vi "Drive.vi"() -> ()   [LabVIEW 2012]
uses:
  State_Machine_Enum.ctl
  <vilib>/Rock Robotics/WPI/RobotDrive/WPI_RobotDriveGetSetRefNum.vi
  Robot Global Data.vi
panel:
  out "Loop Difference":u32
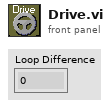
[diagram p1: front panel]
types:
  T1 = typedef "State_Machine_Enum.ctl" = enum16{"Idle", "Start", "Do", "Stop", "Init"}
  T2 = typedef "WPI_RobotDriveDevRef.ctl" = cluster{"DevStatus":errorcluster, "Motors[]":T3[], "Square Inputs":bool, "Max Output":dbl, "Isochronous":bool}
  T3 = typedef "WPI_MotorControlDeviceRef.ctl" = cluster{"DeviceStatus":errorcluster, "Type":enum16{"PWM", "CAN"}, "PWM":cluster{"Digital Module":T4, "PWM Channel":T5, "DeadBand":T6}, "CAN":cluster{"Device Number":u8, "Control Mode":T7, "Semaphore":T8, "Max Vout":dbl}, "Invert":bool, "TransformRef":T9, "InvTransformRef":T9}
  T4 = typedef "FPGA_TypedefDigitalModule.ctl" = enum16{"Digital Module 1", "Digital Module 2"}
  T5 = typedef "FPGA_DIOPWMChannel.ctl" = enum8{"PWM 1", "PWM 2", "PWM 3", "PWM 4", "PWM 5", "PWM 6", "PWM 7", "PWM 8", "PWM 9", "PWM 10", "Invalid"}
  T6 = typedef "WPI_PWMDeadband.ctl" = cluster{"Name":string, "maxPositivePwm":i32, "minPositivePwm":i32, "centerPwm":i32, "maxNegativePwm":i32, "minNegativePwm":i32, "angularRange":u16}
  T7 = typedef "WPI_CANJaguar_ControlMode.ctl" = enum8{"Percent VBus", "Current", "Speed", "Position", "Voltage"}
  T8 = typedef "Semaphore RefNum" = refnum<k1>
  T9 = typedef "WPI_PWMTransform_ConPane.ctl" = refnum<vi>
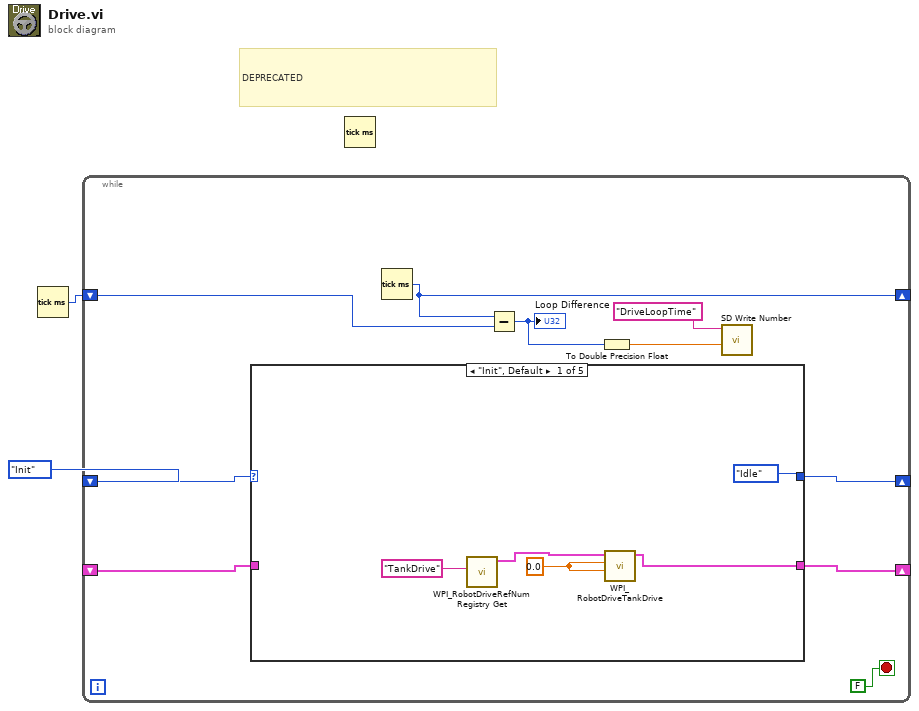
[diagram p0: block diagram]
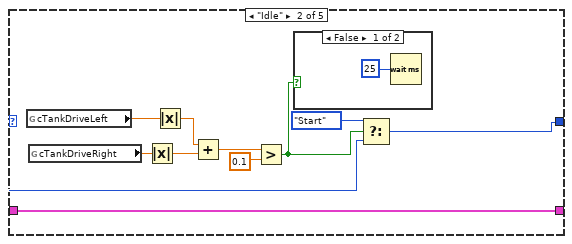
[diagram p2: hidden frame]
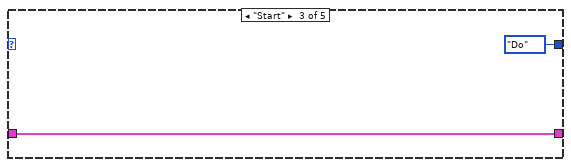
[diagram p4: hidden frame]
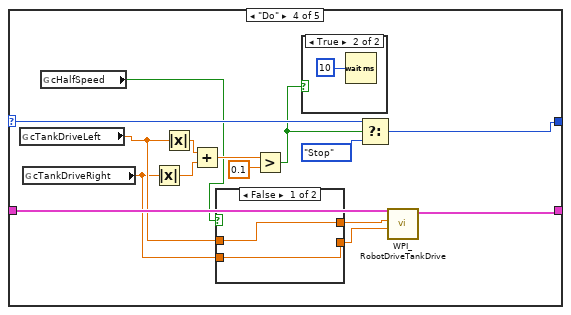
[diagram p5: hidden frame]
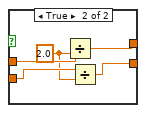
[diagram p6: hidden frame]
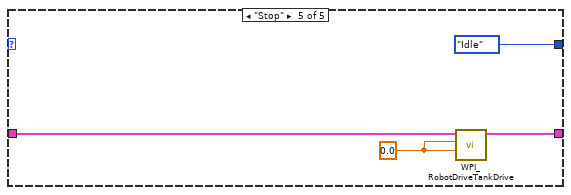
[diagram p8: hidden frame]
diagram:
  # "DEPRECATED"
  n1 = Tick Count (ms)() -> (millisecond timer value=w1:u32)
  n2 = while {
    shift-right: [w11] -> _
    shift-left: State_Machine_Enum."Init" ("State") -> [w12]
    shift-right: [w10] -> _
    shift-left: _ -> [w9]
    shift-right: [w7] -> _
    shift-left: w1 -> [w8]
    stop <- FALSE stop-if-true
    n3 = case shown="\"Init\", Default" w12 {
      selector: w12 -> [_ w23 _ w42 _]
      tunnel: [State_Machine_Enum."Idle" ("State") w22 State_Machine_Enum."Do" ("State") w41 State_Machine_Enum."Idle" ("State")] -> w11
      tunnel: [w14 w18 w31 w40 w57] -> w10
      tunnel: w9 -> [_ w18 w31 w37 w56]
      frame "Init", Default {
        w15 = 0.0 ("Left axis value")
        n4 = call <vilib>:"WPI_RobotDriveRefNum Registry Get.vi"("refnum name"="TankDrive") -> ("RobotDriveDevRef"=w13:T2)  [unwired: 9 in, 1 out]
        n5 = call <vilib>:"WPI_RobotDriveTankDrive.vi"("Right axis value"=w15, "Left axis value"=w15, "RobotDriveDevRef"=w13) -> ("RobotDriveDevRef"=w14:T2)  [unwired: 6 in, 2 out]
      }
      frame "Idle" {
        n6 = global read "Robot Global Data.vi" "cTankDriveLeft"() -> (w21:dbl)
        n7 = global read "Robot Global Data.vi" "cTankDriveRight"() -> (w20:dbl)
        n8 = Absolute Value(x=w20) -> (abs(x)=w27:dbl)
        n9 = Absolute Value(x=w21) -> (abs(x)=w28:dbl)
        n10 = Add(x=w28, y=w27) -> (x+y=w26:dbl)
        n11 = Greater?(x=w26, y=0.1) -> (0:w24:bool)
        n12 = case shown="False" w24 {
          frame False {
            n13 = Wait (ms)(milliseconds to wait=u32 25) -> ()  [unwired: 1 out]
          }
          frame True {
          }
        }
        n14 = Select(t=State_Machine_Enum."Start" ("State"), s=w24, f=w23) -> (s? t:f=w22:T1)
      }
      frame "Start" {
      }
      frame "Do" {
        n15 = global read "Robot Global Data.vi" "cTankDriveLeft"() -> (w36:dbl)
        n16 = global read "Robot Global Data.vi" "cTankDriveRight"() -> (w35:dbl)
        n17 = global read "Robot Global Data.vi" "cHalfSpeed"() -> (w32:bool)
        n18 = Absolute Value(x=w35) -> (abs(x)=w45:dbl)
        n19 = Absolute Value(x=w36) -> (abs(x)=w46:dbl)
        n20 = Add(x=w46, y=w45) -> (x+y=w43:dbl)
        n21 = case shown="False" w32 {
          tunnel: w36 -> [w48 w53]
          tunnel: w35 -> [w47 w52]
          tunnel: [w48 w50] -> w33
          tunnel: [w47 w49] -> w34
          frame False {
          }
          frame True {
            w51 = 2.0 ("y")
            n22 = Divide(x=w53, y=w51) -> (x/y=w50:dbl)
            n23 = Divide(x=w52, y=w51) -> (x/y=w49:dbl)
          }
        }
        n24 = Greater?(x=w43, y=0.1) -> (0:w39:bool)
        n25 = case shown="True" w39 {
          frame False {
          }
          frame True {
            n26 = Wait (ms)(milliseconds to wait=u32 10) -> ()  [unwired: 1 out]
          }
        }
        n27 = Select(t=w42, s=w39, f=State_Machine_Enum."Stop" ("State")) -> (s? t:f=w41:T1)
        n28 = call <vilib>:"WPI_RobotDriveTankDrive.vi"("Right axis value"=w34, "Left axis value"=w33, "RobotDriveDevRef"=w37) -> ("RobotDriveDevRef"=w40:T2)  [unwired: 6 in, 2 out]
      }
      frame "Stop" {
        w58 = 0.0 ("Left axis value")
        n29 = call <vilib>:"WPI_RobotDriveTankDrive.vi"("Right axis value"=w58, "Left axis value"=w58, "RobotDriveDevRef"=w56) -> ("RobotDriveDevRef"=w57:T2)  [unwired: 6 in, 2 out]
      }
    }
    n30 = Tick Count (ms)() -> (millisecond timer value=w7:u32)
    n31 = Subtract(x=w7, y=w8) -> (x-y=w5:u32)
    "Loop Difference" <- w5
    n32 = To Double Precision Float(number=w5) -> (double precision float=w4:dbl)
    n33 = call <vilib>:"SD Write Number.vi"("Numeric"=w4, "Name"="DriveLoopTime") -> ()  [unwired: 8 in, 2 out]
  }
  n34 = Tick Count (ms)() -> ()  [unwired: 1 out]
